vi "LEP_RV_WriteAllSymbolsToXML.vi"(1 "error in":errorcluster, 2 "Sorted objects' names array":string[](array[string]), 3 "Data value reference for\nLabVIEW.map file's lines array":refnum<data-value>, 4 "XML File Refnum":refnum<file>) -> (0 "error out":errorcluster)   [LabVIEW 2011]
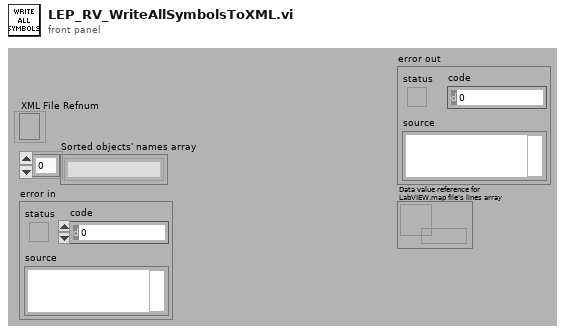
[diagram p1: front panel]
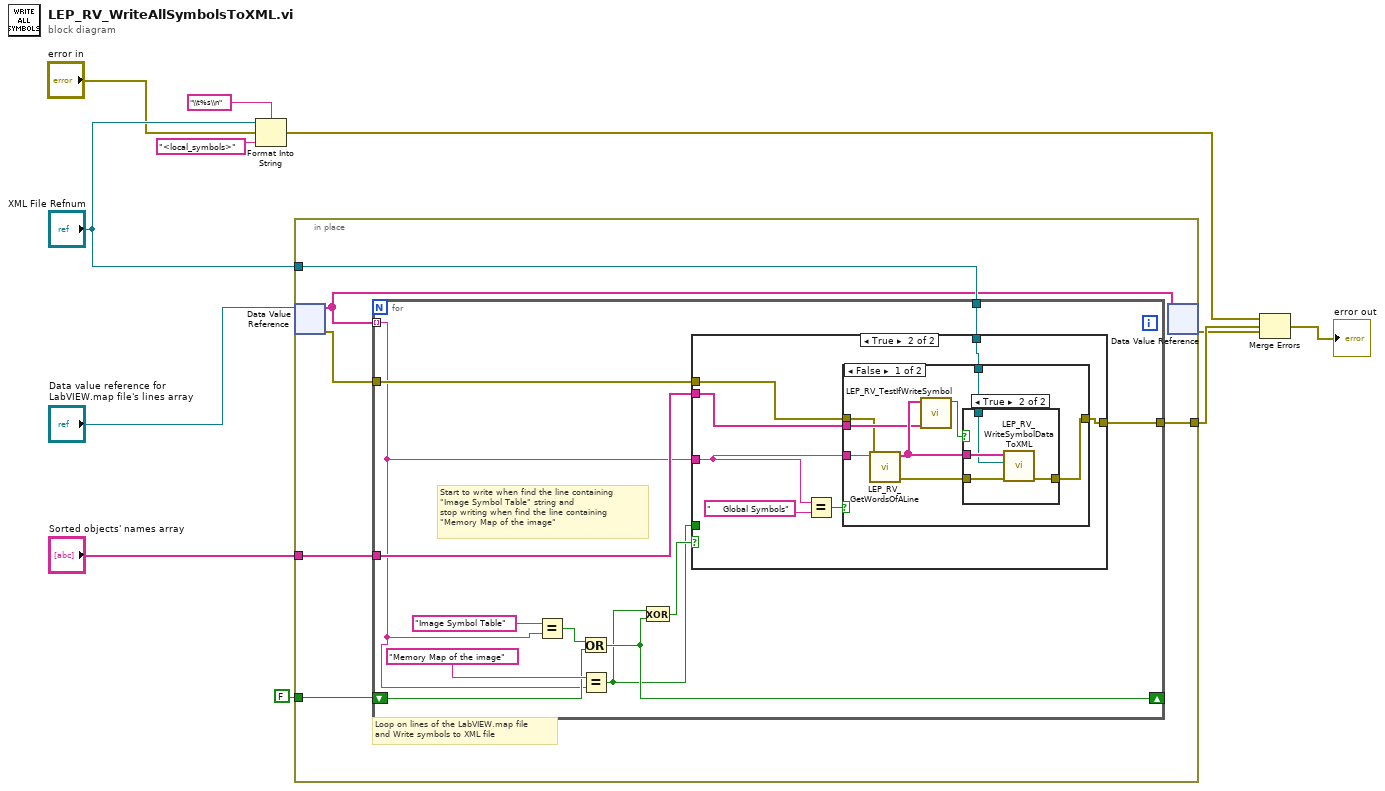
[diagram p0: block diagram]
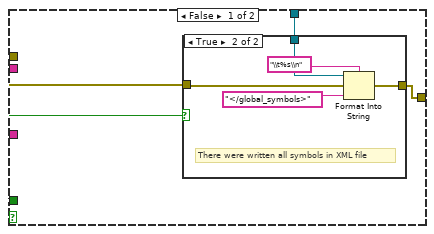
[diagram p2: hidden frame]
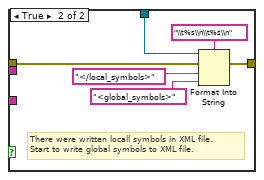
[diagram p5: hidden frame]
diagram:
  n1 = Format Into String(format string="\\t%s\\n", initial string="XML File Refnum", error in="error in", "<local_symbols>" ("input 1")) -> (error out=w4:errorcluster)  [unwired: 1 out]
  n2 = in-place {
    in-place-border: "Sorted objects' names array" -> [w17]
    in-place-border: "XML File Refnum" -> [w16]
    in-place-border: [w15] -> w3
    in-place-border: FALSE -> [w14]
    # "Loop on lines of the LabVIEW.map file\nand Write symbols to XML file"
    n3 = in-place-dvr #1("Data value reference for\nLabVIEW.map file's lines array") -> (w12:string[], w13:errorcluster)
    n4 = for {
      tunnel: w13 -> [w25]
      tunnel: [w24] -> w15
      shift-right: [w22] -> _
      shift-left: w14 -> [w23]
      tunnel: w17 -> [w20]
      tunnel: w12 -> [w19] mode=indexing
      tunnel: w16 -> [w18]
      # "Start to write when find the line containing \n\"Image Symbol Table\" string and\nstop writing when find the line containing \n\"Memory Map of the image\""
      n5 = Equal?(x="Image Symbol Table", y=w19) -> (x = y?=w27:bool)
      n6 = Or(x=w27, y=w23) -> (x .or. y?=w22:bool)
      n7 = Equal?(x="Memory Map of the image" ("substring"), y=w19) -> (x = y?=w21:bool)
      n8 = Exclusive Or(1:w22, 2:w21) -> (0:w26:bool)
      n9 = case shown="True" w26 {
        tunnel: w19 -> [_ w44]
        tunnel: w25 -> [w33 w42]
        tunnel: [w31 w43] -> w24
        tunnel: w21 -> [w32 _]
        tunnel: w20 -> [_ w41]
        tunnel: w18 -> [w30 w40]
        frame False {
          n10 = case shown="True" w32 {
            tunnel: w33 -> [w34 w39]
            tunnel: [w34 w36] -> w31
            tunnel: w30 -> [_ w35]
            frame False {
            }
            frame True {
              # "There were written all symbols in XML file"
              n11 = Format Into String(format string="\\t%s\\n", initial string=w35, error in=w39, "</global_symbols>" ("input 1")) -> (error out=w36:errorcluster)  [unwired: 1 out]
            }
          }
        }
        frame True {
          n12 = Equal?(x=w44, y="    Global Symbols") -> (x = y?=w45:bool)
          n13 = case shown="False" w45 {
            tunnel: w42 -> [w48 w60]
            tunnel: w44 -> [w54 _]
            tunnel: [w51 w62] -> w43
            tunnel: w41 -> [w49 _]
            tunnel: w40 -> [w47 w61]
            frame False {
              n14 = call "LEP_RV_GetWordsOfALine.vi"("error out"=w48, "Initial String"=w54) -> ("error IO"=w52:errorcluster, "Array containing the words (tokens) of a string"=w50:string[])  [unwired: 8 in]
              n15 = call "LEP_RV_TestIfWriteSymbol.vi"("Array with names of objects"=w49, "Symbol's components array"=w50) -> ("Write ?"=w53:bool)  [unwired: 9 in]
              n16 = case shown="True" w53 {
                tunnel: w52 -> [w55 w58]
                tunnel: [w55 w57] -> w51
                tunnel: w50 -> [_ w59]
                tunnel: w47 -> [_ w56]
                frame False {
                }
                frame True {
                  n17 = call "LEP_RV_WriteSymbolDataToXML.vi"("error in"=w58, "XML file refnum"=w56, "Symbol elements array"=w59) -> ("error out"=w57:errorcluster)  [unwired: 8 in]
                }
              }
            }
            frame True {
              # "There were written locall symbols in XML file.\nStart to write global symbols to XML file."
              n18 = Format Into String(format string="\\t%s\\n\\t%s\\n", initial string=w61, error in=w60, "</local_symbols>" ("input 1"), "<global_symbols>" ("input 2")) -> (error out=w62:errorcluster)  [unwired: 1 out]
            }
          }
        }
      }
    }
    n19 = in-place-dvr #1(w12) -> (w2:errorcluster)  [unwired: 1 out]
  }
  n20 = Merge Errors(w4, w3, w2) -> (→"error out":errorcluster)
